vi "SetObjectConfigurationString.vi"(8 "ErrorIn":errorcluster, 9 "String":string, 10 "Label":string, 11 "ReferenceIn":refnum<class "AppConfigJSON.lvclass">) -> (0 "ErrorOut":errorcluster, 3 "ReferenceOut":refnum<class "AppConfigJSON.lvclass">)   [LabVIEW 2021, in "AppConfigJSON.lvclass"]
uses:
  AppConfigJSON.lvclass
  <vilib>/JDP Science/JSONtext/Config Files/Config File.lvclass/Config File.ctl
  <vilib>/JDP Science/JSONtext/Config Files/Write Config to File.vi
  AppConfigJSON.lvclass/AppConfigJSON.ctl
  <vilib>/JDP Science/JSONtext/Config Files/Config File.lvclass
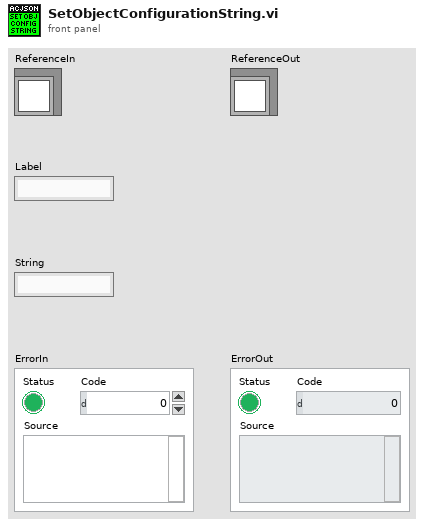
[diagram p1: front panel]
types:
  T1 = typedef "AppConfigJSON.lvclass/ObjectAttributes.ctl" = cluster{"Name":string, "ConfigFilePath":path, "Objects":T2[], "ApplicationBasePath":path, "ObjectName":string}
  T2 = typedef "IApplicationConfiguration.lvclass/ObjectDataDetails.ctl" = cluster{"ObjectName":string, "ObjectType":string, "Interfaces":T3[]}
  T3 = typedef "IApplicationConfiguration.lvclass/ObjectData.ctl" = cluster{"Label":string, "ObjectName":string, "Type":string}
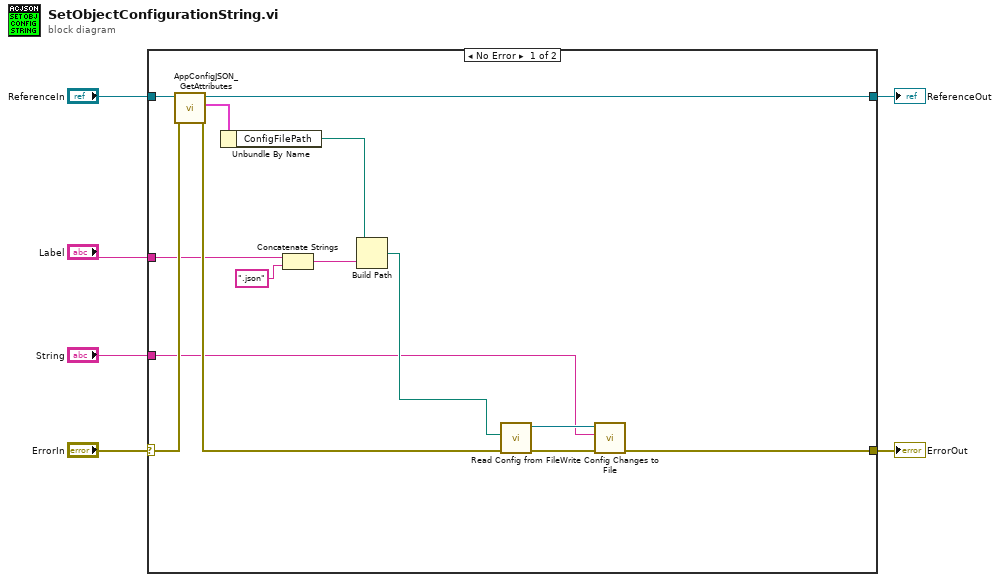
[diagram p0: block diagram]
diagram:
  n1 = case shown="No Error" "ErrorIn" {
    selector: "ErrorIn" -> [w20 w22]
    tunnel: [w18 w22] -> w5
    tunnel: [w14 w21] -> w3
    tunnel: "ReferenceIn" -> [w15 w21]
    tunnel: "Label" -> [w12 _]
    tunnel: "String" -> [w7 _]
    frame No Error {
      n2 = call "AppConfigJSON_GetAttributes.vi"("ErrorIn"=w20, "ReferenceIn"=w15) -> ("ErrorOut"=w19:errorcluster, "Data"=w16:T1, "ReferenceOut"=w14:refnum<class "AppConfigJSON.lvclass">)  [unwired: 6 in, 1 out]
      n3 = Unbundle By Name(w16) -> ("ConfigFilePath"=w13:path)
      n4 = Concatenate Strings(w12, ".json" ("string")) -> (w10:string)
      n5 = Build Path(base path=w13, name or relative path=w10) -> (appended path=w11:path)
      n6 = call <vilib>:"Read Config from File.vi"("error in (no error)"=w19, "config file path"=w11) -> ("error out"=w17:errorcluster, "Config File"=w8:refnum<class "Config File.lvclass">)  [unwired: 6 in, 2 out]
      n7 = call <vilib>:"Write Config Changes to File.vi"("error in (no error)"=w17, "New Config"=w7, "Config File in"=w8) -> ("error out"=w18:errorcluster)  [unwired: 5 in, 3 out]
    }
    frame Error {
    }
  }
  "ErrorOut" <- w5
  "ReferenceOut" <- w3
